vi "Wait at Rendezvous.vi"(4 "error in (no error)":errorcluster, 5 "ms timeout (-1)":i32=-1, 7 "rendezvous":T1) -> (0 "error out":errorcluster, 1 "timed out":bool, 3 "rendezvous out":T1)   [LabVIEW 2020]
doc: "Waits until a sufficient number of tasks have arrived at the rendezvous."
uses:
  RendezvousDataCluster.ctl
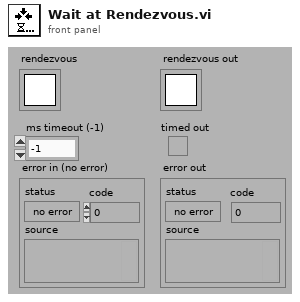
[diagram p1: front panel]
types:
  T1 = typedef "Rendezvous RefNum" = refnum<k1>
  T2 = typedef "RendezvousDataCluster.ctl" = cluster{"Threshold":i32, "Messenger Queues":refnum<queue>[]}
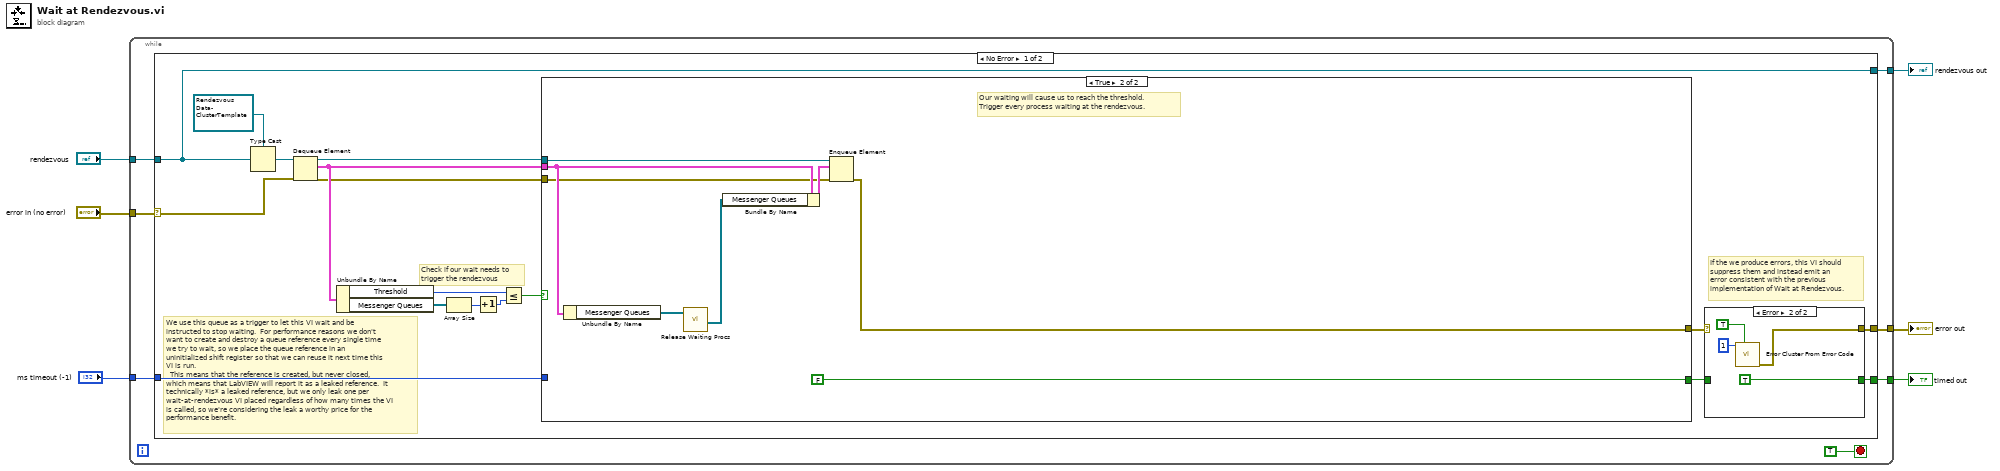
[diagram p0: block diagram]
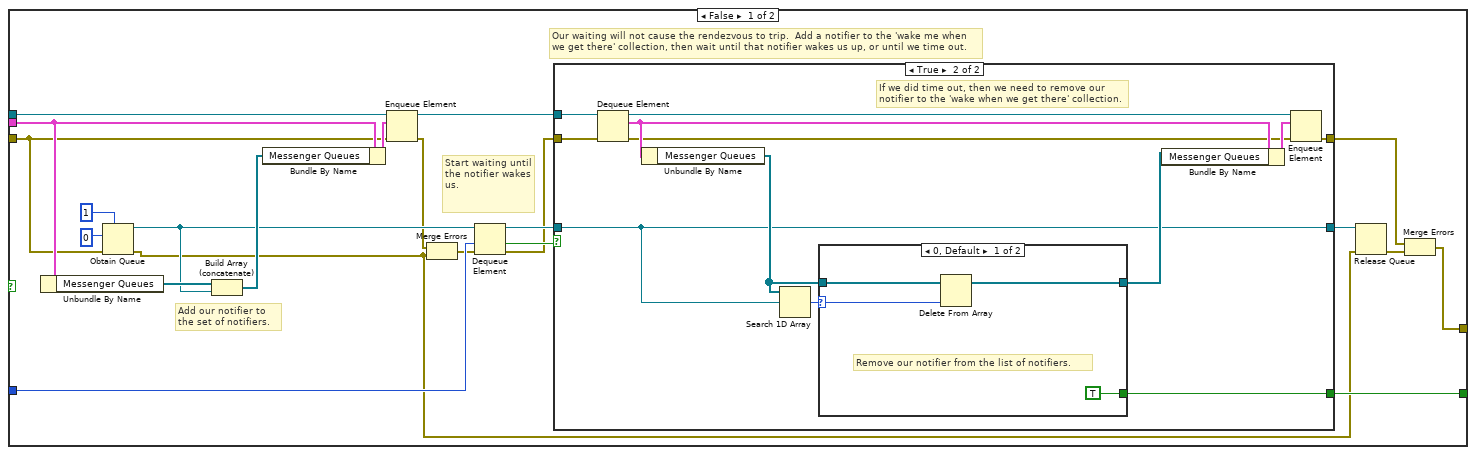
[diagram p2: hidden frame]
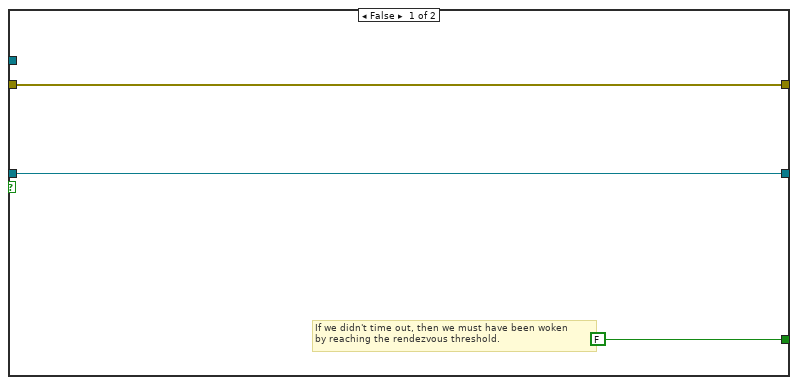
[diagram p3: hidden frame]
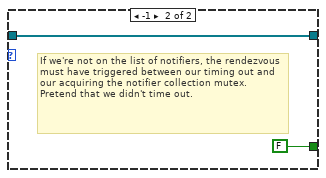
[diagram p4: hidden frame]
diagram:
  n1 = while {
    tunnel: [w13] -> w6
    tunnel: [w12] -> w5
    tunnel: "rendezvous" -> [w11]
    tunnel: [w10] -> w3
    tunnel: "error in (no error)" -> [w9]
    tunnel: "ms timeout (-1)" -> [w8]
    stop <- TRUE stop-if-true
    n2 = case shown="No Error" w9 {
      selector: w9 -> [w17 w90]
      tunnel: [w30 w90] -> w13
      tunnel: [w29 FALSE] -> w12
      tunnel: w11 -> [w15 w89]
      tunnel: [w15 w89] -> w10
      tunnel: w8 -> [w23 _]
      frame No Error {
        # "We use this queue as a trigger to let this VI wait and be instructed to stop waiting.  For performance reasons we don't want to create and destroy a queue reference every single time we try to wait, so we place the queue reference in an uninitialized shift register so that we can reuse it next time this VI is run.  \n  This means that the reference is created, but never closed, which means that LabVIEW will report it as a leaked reference.  It technically *is* a leaked reference, but we only leak one per wait-at-rendezvous VI placed regardless of how many times the VI is called, so we're considering the leak a worthy price for the performance benefit."
        # "Check if our wait needs to trigger the rendezvous"
        # "If the we produce errors, this VI should suppress them and instead emit an error consistent with the previous implementation of Wait at Rendezvous."
        n3 = Type Cast(type=refnum<queue> refnum ("queue out"), x=w15) -> (*(type *) &x=w16:refnum<queue>)
        n4 = Dequeue Element(queue=w16, error in (no error)=w17) -> (queue out=w25:refnum<queue>, element=w21:T2, error out=w19:errorcluster)  [unwired: 2 out]
        n5 = Unbundle By Name(w21) -> ("Threshold"=w27:i32, "Messenger Queues"=w18:refnum<queue>[])
        n6 = Array Size(array=w18) -> (size(s)=w20:i32)
        n7 = Increment(x=w20) -> (x+1=w28:i32)
        n8 = Less Or Equal?(x=w27, y=w28) -> (x <= y?=w26:bool)
        n9 = case shown="True" w26 {
          tunnel: [w31 w79] -> w24
          tunnel: w25 -> [w51 w80]
          tunnel: w23 -> [w50 _]
          tunnel: [w52 FALSE] -> w22
          tunnel: w21 -> [w45 w75]
          tunnel: w19 -> [w39 w74]
          frame False {
            # "Start waiting until the notifier wakes us."
            # "Add our notifier to the set of notifiers."
            # "Our waiting will not cause the rendezvous to trip.  Add a notifier to the 'wake me when we get there' collection, then wait until that notifier wakes us up, or until we time out."
            n10 = Unbundle By Name(w45) -> ("Messenger Queues"=w44:refnum<queue>[])
            n11 = Obtain Queue(max queue size (-1, unlimited)=1, element data type=0, error in (no error)=w39) -> (queue out=w40:refnum<queue>, error out=w35:errorcluster)  [unwired: 1 in, 2 out]
            n12 = Build Array (concatenate)(w44, w40) -> (w43:refnum<queue>[])
            n13 = Bundle By Name(cluster=w45, "Messenger Queues"=w43) -> (w49:T2)
            n14 = Enqueue Element(queue=w51, element=w49, error in (no error)=w39) -> (queue out=w48:refnum<queue>, error out=w38:errorcluster)  [unwired: 2 out]
            n15 = Merge Errors(w38, w35) -> (w37:errorcluster)
            n16 = Dequeue Element(queue=w40, timeout in ms (-1)=w50, error in (no error)=w37) -> (queue out=w46:refnum<queue>, timed out?=w47:bool, error out=w34:errorcluster)  [unwired: 1 out]
            n17 = case shown="True" w47 {
              tunnel: [w54 w62] -> w33
              tunnel: [FALSE w66] -> w52
              tunnel: w48 -> [_ w65]
              tunnel: w34 -> [w54 w64]
              tunnel: w46 -> [w53 w56]
              tunnel: [w53 w56] -> w36
              frame False {
                # "If we didn't time out, then we must have been woken\nby reaching the rendezvous threshold."
              }
              frame True {
                # "If we did time out, then we need to remove our notifier to the 'wake when we get there' collection."
                n18 = Dequeue Element(queue=w65, error in (no error)=w64) -> (queue out=w63:refnum<queue>, element=w60:T2, error out=w57:errorcluster)  [unwired: 2 out]
                n19 = Unbundle By Name(w60) -> ("Messenger Queues"=w61:refnum<queue>[])
                n20 = Search 1D Array(1D array=w61, element=w56) -> (index of element=w67:i32)  [unwired: 1 out]
                n21 = case shown="0, Default" w67 {
                  selector: w67 -> [w71 _]
                  tunnel: [w70 w72] -> w58
                  tunnel: [TRUE FALSE] -> w66
                  tunnel: w61 -> [w68 w72]
                  frame 0, Default {
                    # "Remove our notifier from the list of notifiers."
                    n22 = Delete From Array(array=w68, index=w71) -> (array with subset deleted=w70:refnum<queue>[])  [unwired: 1 in, 1 out]
                  }
                  frame -1 {
                    # "If we're not on the list of notifiers, the rendezvous must have triggered between our timing out and our acquiring the notifier collection mutex.  Pretend that we didn't time out."
                  }
                }
                n23 = Bundle By Name(cluster=w60, "Messenger Queues"=w58) -> (w59:T2)
                n24 = Enqueue Element(queue=w63, element=w59, error in (no error)=w57) -> (error out=w62:errorcluster)  [unwired: 3 out]
              }
            }
            n25 = Release Queue(queue=w36, error in (no error)=w35) -> (error out=w32:errorcluster)  [unwired: 1 in, 2 out]
            n26 = Merge Errors(w33, w32) -> (w31:errorcluster)
          }
          frame True {
            # "Our waiting will cause us to reach the threshold.\nTrigger every process waiting at the rendezvous."
            n27 = Unbundle By Name(w75) -> ("Messenger Queues"=w76:refnum<queue>[])
            n28 = call "Release Waiting Procs.vi"("Notifiers"=w76) -> ("Notifiers Out"=w77:refnum<queue>[])  [unwired: 2 in, 8 out]
            n29 = Bundle By Name(cluster=w75, "Messenger Queues"=w77) -> (w78:T2)
            n30 = Enqueue Element(queue=w80, element=w78, error in (no error)=w74) -> (error out=w79:errorcluster)  [unwired: 3 out]
          }
        }
        n31 = case shown="Error" w24 {
          selector: w24 -> [w83 _]
          tunnel: [w83 w87] -> w30
          tunnel: [w82 TRUE] -> w29
          tunnel: w22 -> [w82 _]
          frame No Error {
          }
          frame Error {
            n32 = call "Error Cluster From Error Code.vi"("show call chain? (False)"=TRUE, "error code (0)"=1) -> ("error out"=w87:errorcluster)  [unwired: 1 in, 6 out]
          }
        }
      }
      frame Error {
        # "If there was an error, do not interact\nwith the rendezvous at all."
      }
    }
  }
  "rendezvous out" <- w3
  "error out" <- w6
  "timed out" <- w5
